vi "Login2.vi"() -> ()   [LabVIEW 2020]
panel:
  in  "Login":bool
  in  "Reset":bool
  in  "Password":string
  in  "User Name":string
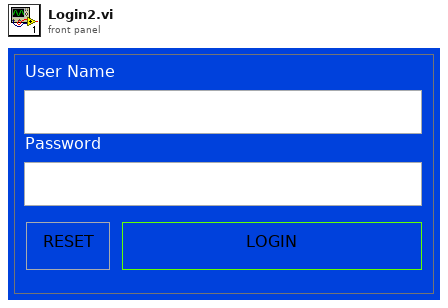
[diagram p1: front panel]
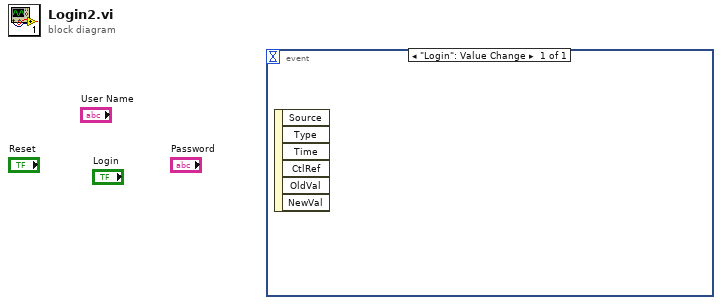
[diagram p0: block diagram]
diagram:
  n1 = event shown="[0] \"Login\": Value Change" {
    selector: _ -> [_]
    dyn-events: _ -> [_]
    timeout: _ -> [_]
    event "Login": Value Change {
      n2 = event-data() -> ()  [unwired: 1 in, 6 out]
    }
  }
